vi "zmq proxy steerable.vi"(0 "frontend_":u32, 5 "backend_":u32, 7 "capture_":u32, 9 "control_":u32, 11 "error in (no error)":errorcluster) -> (3 "function return":i32, 4 "frontend_ out":u32, 6 "backend_ out":u32, 8 "capture_ out":u32, 10 "control_ out":u32, 15 "error out":errorcluster)   [LabVIEW 2025, in "libzmq-v143-mt-4_3_6.lvlib"]
doc: "ZMQ_EXPORT int zmq_proxy_steerable (void *frontend_,\n void *backend_,\n void *capture_,\n void *control_);"
uses:
  libzmq-v143-mt-4_3_6.lvlib
  LV/LibZMQ/libzmq/lv_x86/bin/Release/libzmq-v143-mt-4_3_6.dll
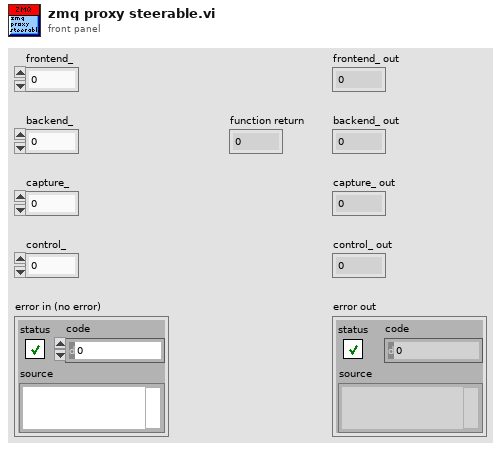
[diagram p1: front panel]
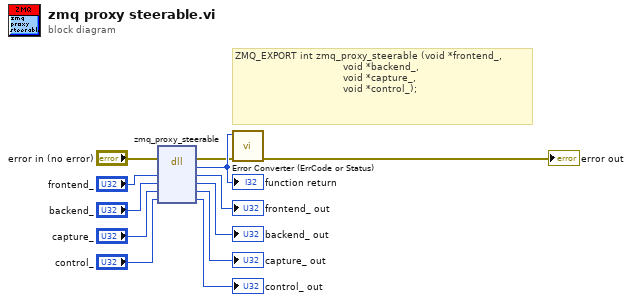
[diagram p0: block diagram]
diagram:
  # "ZMQ_EXPORT int zmq_proxy_steerable (void *frontend_,\n                                    void *backend_,\n                                    void *capture_,\n                                    void *control_);"
  n1 = dll-call lib="C:/LV/LibZMQ/libzmq/lv_x86/bin/Release/libzmq-v143-mt-4_3_6.*" fn="zmq_proxy_steerable"(error in="error in (no error)", "frontend_"="frontend_", "backend_"="backend_", "capture_"="capture_", "control_"="control_") -> (error out=w2:errorcluster, w12:i32, "frontend_"=→"frontend_ out":u32, "backend_"=→"backend_ out":u32, "capture_"=→"capture_ out":u32, "control_"=→"control_ out":u32)  [unwired: 2 in, 1 out]
  "function return" <- w12
  n2 = call "Error Converter (ErrCode or Status).vi"("error in (no error)"=w2, "error code"=w12) -> ("error out"=→"error out":errorcluster)  [unwired: 9 in]
